vi "Name.vi"(8 "error in (no error)":errorcluster, 11 "Test Suite with Global Fixture In":refnum<class "Test Suite with Global Fixture.lvclass">) -> (0 "error out":errorcluster, 2 "Name":string, 3 "Test Suite with Global Fixture Out":refnum<class "Test Suite with Global Fixture.lvclass">)   [LabVIEW 2020, in "Test Suite with Global Fixture.lvclass"]
uses:
  Test Suite with Global Fixture.lvclass
  Test Suite with Global Fixture.lvclass/Test Suite with Global Fixture.ctl
  <vilib>/Astemes/LUnit/Test Suite.lvclass
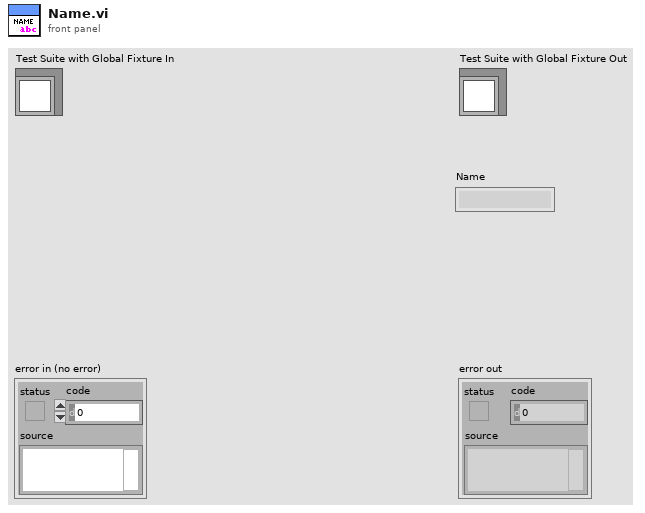
[diagram p1: front panel]
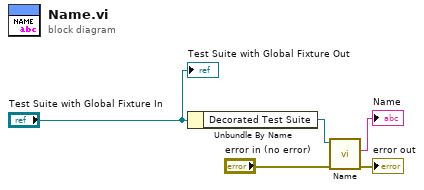
[diagram p0: block diagram]
diagram:
  n1 = Unbundle By Name("Test Suite with Global Fixture In") -> ("Decorated Test Suite"=w4:refnum<class "Test Suite.lvclass">)
  n2 = call-dynamic "Name.vi"("error in (no error)"="error in (no error)", "LUnit Test Suite in"=w4) -> ("error out"=→"error out":errorcluster, "Name"=→"Name":string)  [unwired: 7 in, 1 out]
  "Test Suite with Global Fixture Out" <- "Test Suite with Global Fixture In"
